vi "Display wave_Cypher.vi"() -> ()   [LabVIEW 2019]
doc: "This Vi only displays 'XMove' 'YMove' wave (used to do lithography) in Igor.\nThis Vi is used to debug"
panel:
  out "History":string="%fprintf 0, \"%f\",td_ReadValue(\"difference%laser\")\r"
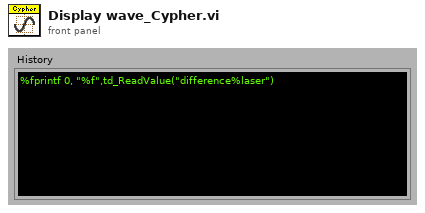
[diagram p1: front panel]
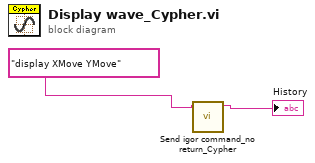
[diagram p0: block diagram]
diagram:
  n1 = call "Send igor command_no return_Cypher.vi"("Command"="display XMove YMove") -> ("History"=→"History":string)  [unwired: 9 in, 1 out]
